vi "Get Picture.vi"(8 "error in (no error)":errorcluster, 11 "Single Cell Battery in":refnum<class "Single Cell Battery.lvclass">) -> (0 "error out":errorcluster, 2 "Picture":picture, 3 "Single Cell Battery out":refnum<class "Single Cell Battery.lvclass">)   [LabVIEW 2020, in "Single Cell Battery.lvclass"]
uses:
  Single Cell Battery.lvclass
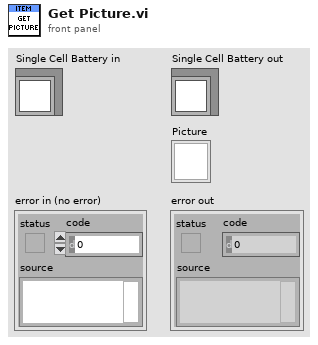
[diagram p1: front panel]
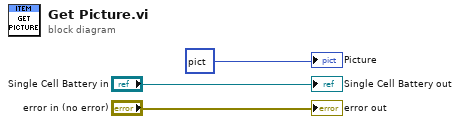
[diagram p0: block diagram]
diagram:
  "error out" <- "error in (no error)"
  "Single Cell Battery out" <- "Single Cell Battery in"
  "Picture" <- picture bytes[3230] ("new picture")
